vi "GEOM_SetExtensionsOrder.vi"(10 "extensions":i32[](array[numeric])) -> (2 "response":string)   [LabVIEW 2016]
uses:
  GEOM_Gbls.vi
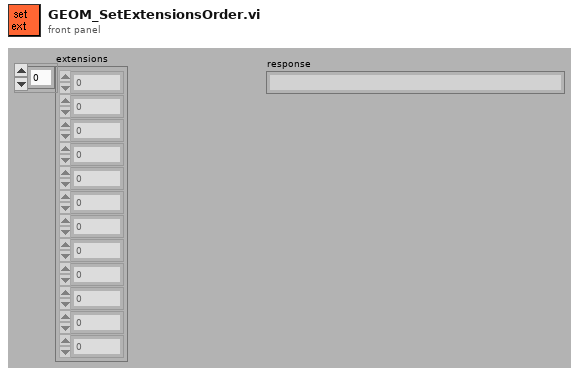
[diagram p1: front panel]
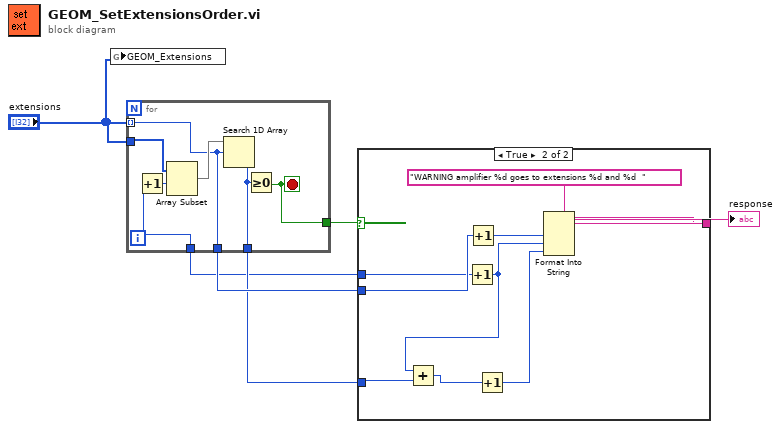
[diagram p0: block diagram]
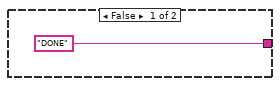
[diagram p2: hidden frame]
diagram:
  n1 = global write "GEOM_Gbls.vi" "GEOM_Extensions"("extensions") -> ()
  n2 = for {
    tunnel: "extensions" -> [w10] mode=indexing
    tunnel: "extensions" -> [w13]
    tunnel: [w11] -> w5
    tunnel: [w10] -> w4
    tunnel: [w9] -> w3
    tunnel: [w8] -> w2
    i -> [w8]
    stop <- w11 stop-if-true
    n3 = Increment(x=w8) -> (x+1=w7:i32)
    n4 = Array Subset(array=w13, index=w7) -> (w12:i32[])  [unwired: 1 in]
    n5 = Search 1D Array(1D array=w12, element=w10) -> (index of element=w9:i32)  [unwired: 1 out]
    n6 = Greater Or Equal To 0?(x=w9) -> (x >= 0?=w11:bool)
  }
  n7 = case shown="True" w5 {
    tunnel: ["DONE" w21] -> w6
    tunnel: w2 -> [_ w16]
    tunnel: w4 -> [_ w22]
    tunnel: w3 -> [_ w18]
    frame False {
    }
    frame True {
      n8 = Increment(x=w16) -> (x+1=w15:i32)
      n9 = Add(x=w15, y=w18) -> (x+y=w17:i32)
      n10 = Increment(x=w22) -> (x+1=w20:i32)
      n11 = Increment(x=w17) -> (x+1=w19:i32)
      n12 = Format Into String(format string="WARNING amplifier %d goes to extensions %d and %d  ", w20, w15, w19) -> (resulting string=w21:string)  [unwired: 2 in, 1 out]
    }
  }
  "response" <- w6
